vi "add_data_line_exp.vi"(8 "error in (no error)":errorcluster, 10 "add Array":dbl[](array[numeric]), 11 "Experiment.lvclass in":refnum<class "Experiment.lvclass">) -> (0 "error out":errorcluster, 3 "Experiment.lvclass out":refnum<class "Experiment.lvclass">)   [LabVIEW 2018, in "Experiment.lvclass"]
uses:
  Experiment.lvclass
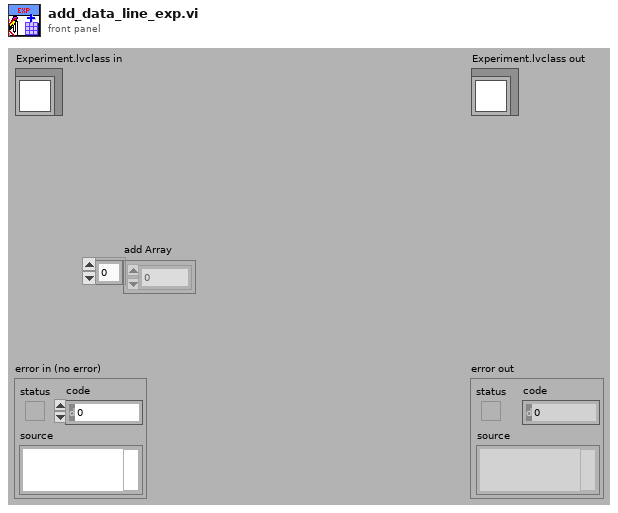
[diagram p1: front panel]
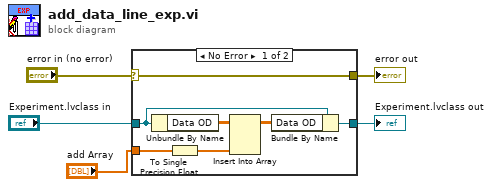
[diagram p0: block diagram]
diagram:
  n1 = case shown="No Error" "error in (no error)" {
    selector: "error in (no error)" -> [w12 w13]
    tunnel: [w12 w13] -> w4
    tunnel: [w11 w14] -> w2
    tunnel: "Experiment.lvclass in" -> [w10 w14]
    tunnel: "add Array" -> [w7 _]
    frame No Error {
      n2 = Unbundle By Name(w10) -> ("Data OD"=w9:sgl[][])
      n3 = To Single Precision Float(number=w7) -> (single precision float=w6:sgl[])
      n4 = Insert Into Array(array=w9, new element=w6) -> (w8:sgl[][])  [unwired: 2 in]
      n5 = Bundle By Name(cluster=w10, "Data OD"=w8) -> (w11:refnum<class "Experiment.lvclass">)
    }
    frame Error {
    }
  }
  "error out" <- w4
  "Experiment.lvclass out" <- w2
